vi "MacrosToTrace_v5.vi"(2 "clocktimePS":i32=50000, 3 "BintimeNS":i32=100000, 4 "Macros":i32[](array[numeric])) -> (0 "counts":i32, 1 "Trace":i32[](array[numeric]))   [LabVIEW 2009]
panel:
  in  "Case Constant\n(See Context Help)":bool=TRUE
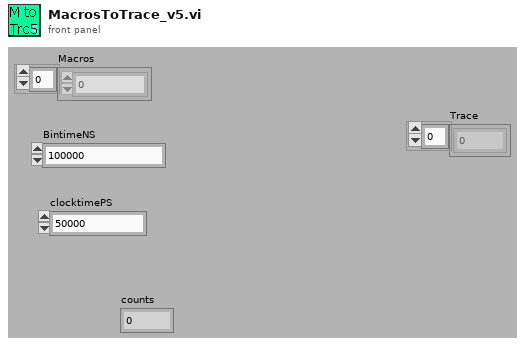
[diagram p1: front panel]
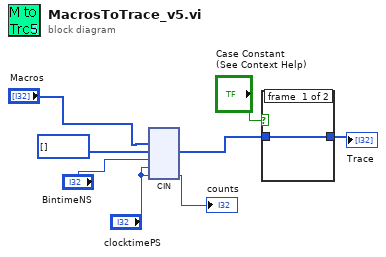
[diagram p0: block diagram]
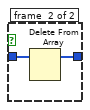
[diagram p2: hidden frame]
diagram:
  n1 = cin("Macros", i32[] [] ("empty"), "BintimeNS", "clocktimePS", "clocktimePS") -> (w3:i32[], →"counts":i32)  [unwired: 3 in]
  n2 = case shown="True" "Case Constant\n(See Context Help)" {
    tunnel: w3 -> [w9 w11]
    tunnel: [w9 w10] -> w2
    frame #0 {
    }
    frame #1 {
      n3 = Delete From Array(array=w11) -> (array with subset deleted=w10:i32[])  [unwired: 2 in, 1 out]
    }
  }
  "Trace" <- w2
